vi "Read Process Action Name.vi"(8 "error in (no error)":errorcluster, 11 "MPC_Laser Marked in":refnum<class "MPC_Laser Marked.lvclass">) -> (0 "error out":errorcluster, 2 "Process Action Name":string[](array[string]), 3 "MPC_Laser Marked out":refnum<class "MPC_Laser Marked.lvclass">)   [LabVIEW 2019, in "MPC_Laser Marked.lvclass"]
uses:
  MPC_Laser Marked.lvclass
  MPC_Laser Marked.lvclass/MPC_Laser Marked.ctl
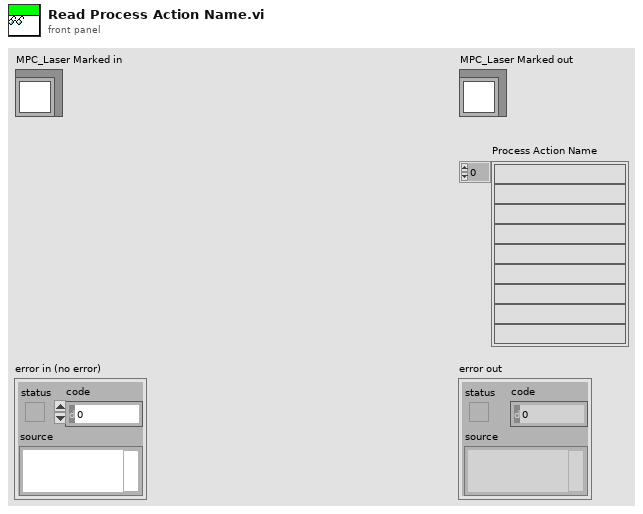
[diagram p1: front panel]
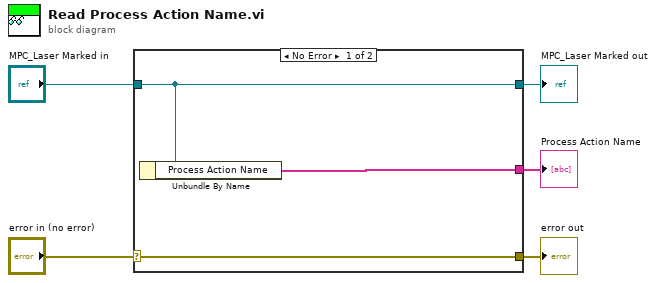
[diagram p0: block diagram]
diagram:
  n1 = case shown="No Error" "error in (no error)" {
    selector: "error in (no error)" -> [w8 w9]
    tunnel: [w8 w9] -> w4
    tunnel: [w7 w10] -> w2
    tunnel: "MPC_Laser Marked in" -> [w7 w10]
    tunnel: [w6 _] -> w1
    frame No Error {
      n2 = Unbundle By Name(w7) -> ("Process Action Name"=w6:string[])
    }
    frame Error {
    }
  }
  "error out" <- w4
  "MPC_Laser Marked out" <- w2
  "Process Action Name" <- w1
